vi "LCD Init by string.vi"(8 "error in":errorcluster, 11 "FPGA VI Reference In":T1) -> (0 "error out":errorcluster, 3 "FPGA VI Reference Out":T1)   [LabVIEW 2019]
uses:
  TypeDefs/FPGA Reference.ctl
  <vilib>/Utility/error.llb/Error Cluster From Error Code.vi
  <vilib>/rvi/errors/niLvFpgaAdjustHostInterfaceError.vi
  <vilib>/rvi/interface/nirviReadWriteControl/nirviReadWriteControl.xnode
  NiFpgaLv.dll
  <vilib>/rvi/interface/Simulation/niFpgaSimulationCallBeginRW.vi
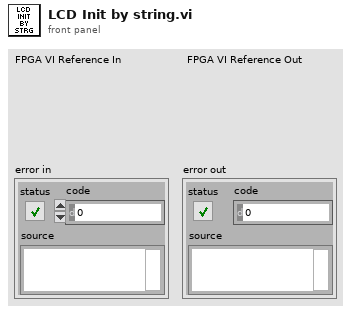
[diagram p1: front panel]
types:
  T1 = typedef "FPGA Reference.ctl" = refnum<k20>
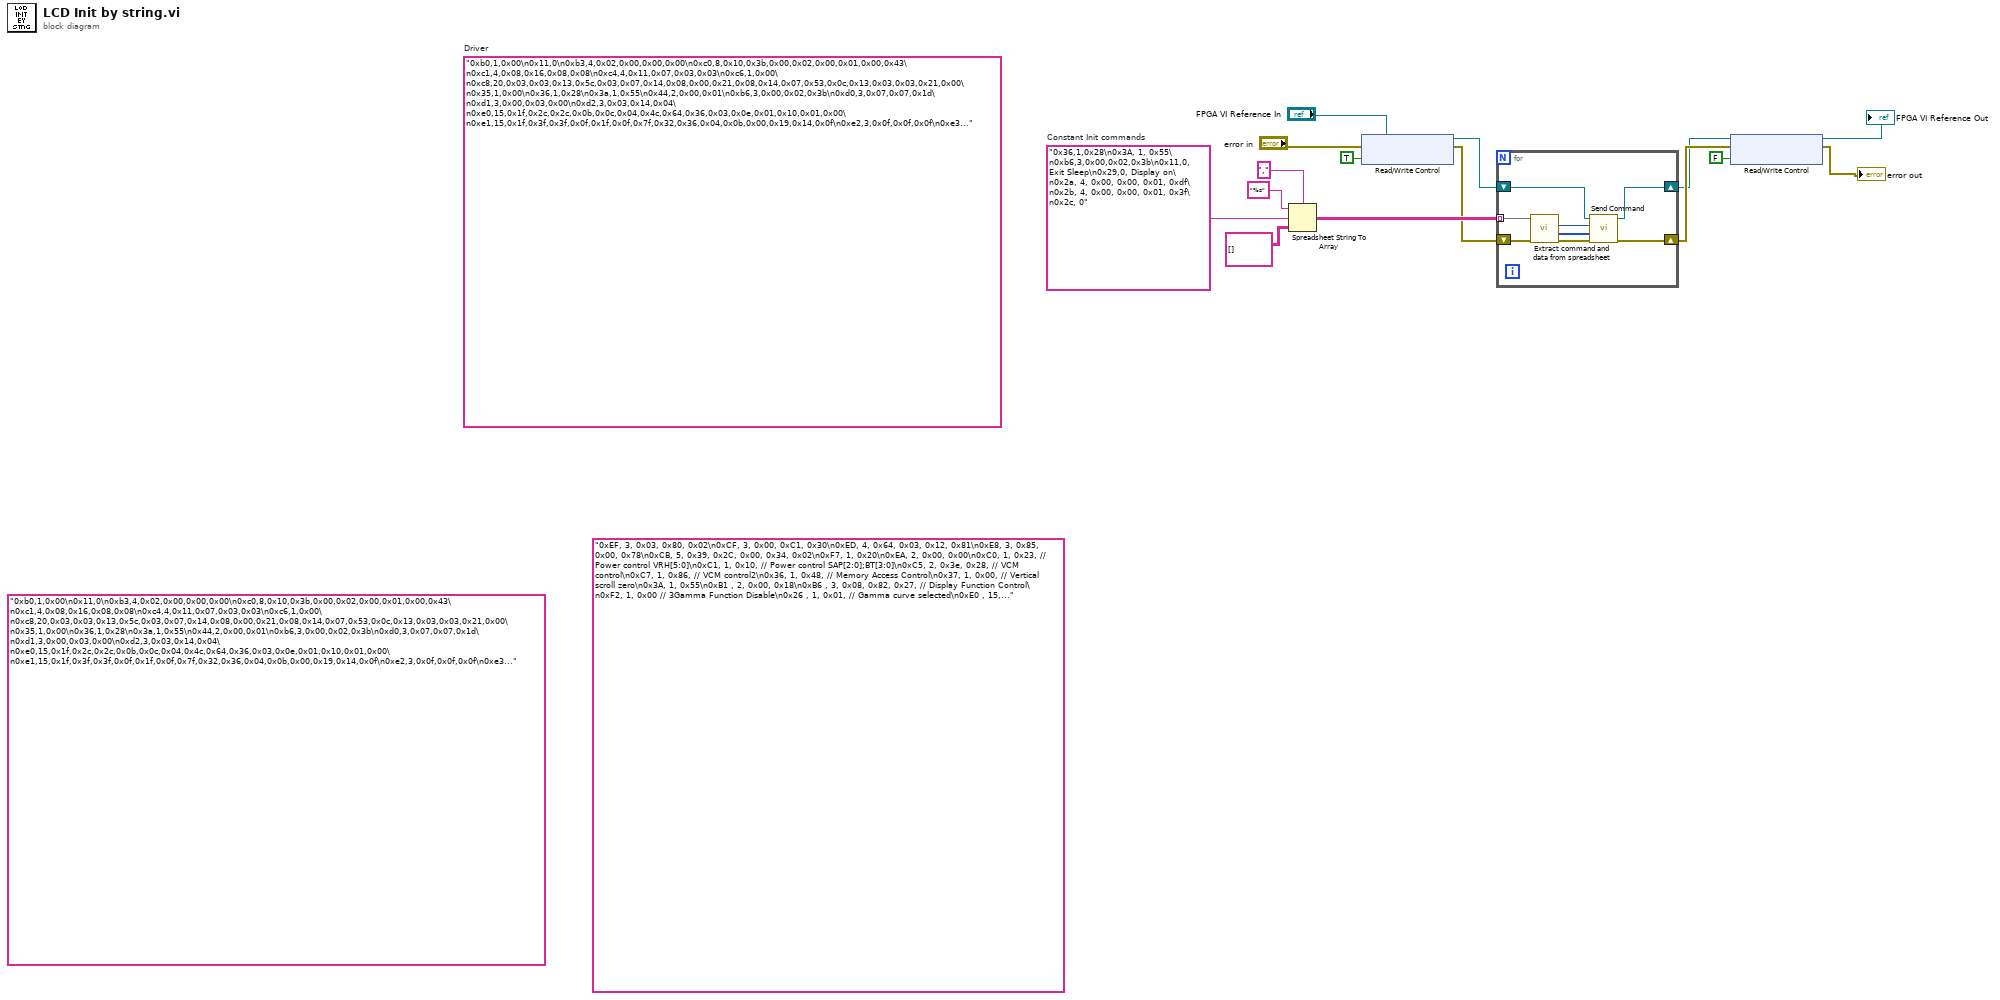
[diagram p0: block diagram]
diagram:
  w11 = "0x36,1,0x28\n0x3A, 1, 0x55\n0xb6,3,0x00,0x02,0x3b\n0x11,0, Exit Sleep\n0x29,0, Display on\n0x2a, 4, 0x00, 0x00, 0x01, 0xdf\n0x2b, 4, 0x00, 0x00, 0x01, 0x3f\n0x2c, 0"  # Constant Init commands
  (unwired) "0xEF, 3, 0x03, 0x80, 0x02\n0xCF, 3, 0x00, 0xC1, 0x30\n0xED, 4, 0x64, 0x03, 0x12, 0x81\n0xE8, 3, 0x85, 0x00, 0x78\n0xCB, 5, 0x39, 0x2C, 0x00, 0x34, 0x02\n0xF7, 1, 0x20\n0xEA, 2, 0x00, 0x00\n0xC0, 1, 0x23, // Power control VRH[5:0]\n0xC1, 1, 0x10, // Power control SAP[2:0];BT[3:0]\n0xC5, 2, 0x3e, 0x28, // VCM control\n0xC7, 1, 0x86, // VCM control2\n0x36, 1, 0x48, // Memory Access Control\n0x37, 1, 0x00, // Vertical scroll zero\n0x3A, 1, 0x55\n0xB1 , 2, 0x00, 0x18\n0xB6 , 3, 0x08, 0x82, 0x27, // Display Function Control\n0xF2, 1, 0x00 // 3Gamma Function Disable\n0x26 , 1, 0x01, // Gamma curve selected\n0xE0 , 15, 0x0F, 0x31, 0x2B, 0x0C, 0x0E, 0x08, 0x4E, 0xF1, 0x37, 0x07, 0x10, 0x03, 0x0E, 0x09, 0x00,\n0xE1 , 15, 0x00, 0x0E, 0x14, 0x03, 0x11, 0x07, 0x31, 0xC1, 0x48, 0x08, 0x0F, 0x0C, 0x31, 0x36, 0x0F\n0x11, 0x80,// Exit Sleep\n0x29, 0x80,// Display on\n0x2a, 4, 0x00, 0x00, 0x01, 0xdf\n0x2b, 4, 0x00, 0x00, 0x01, 0x3f\n0x2c, 0"
  (unwired) "0xb0,1,0x00\n0x11,0\n0xb3,4,0x02,0x00,0x00,0x00\n0xc0,8,0x10,0x3b,0x00,0x02,0x00,0x01,0x00,0x43\n0xc1,4,0x08,0x16,0x08,0x08\n0xc4,4,0x11,0x07,0x03,0x03\n0xc6,1,0x00\n0xc8,20,0x03,0x03,0x13,0x5c,0x03,0x07,0x14,0x08,0x00,0x21,0x08,0x14,0x07,0x53,0x0c,0x13,0x03,0x03,0x21,0x00\n0x35,1,0x00\n0x36,1,0x28\n0x3a,1,0x55\n0x44,2,0x00,0x01\n0xb6,3,0x00,0x02,0x3b\n0xd0,3,0x07,0x07,0x1d\n0xd1,3,0x00,0x03,0x00\n0xd2,3,0x03,0x14,0x04\n0xe0,15,0x1f,0x2c,0x2c,0x0b,0x0c,0x04,0x4c,0x64,0x36,0x03,0x0e,0x01,0x10,0x01,0x00\n0xe1,15,0x1f,0x3f,0x3f,0x0f,0x1f,0x0f,0x7f,0x32,0x36,0x04,0x0b,0x00,0x19,0x14,0x0f\n0xe2,3,0x0f,0x0f,0x0f\n0xe3,3,0x0f,0x0f,0x0f\n0x13,0\n0x29,0\n0xb4,1,0x00\n0x2xc,0\n0x2a,4,0x00,0x00,0x01,0xdf\n0x2b,4,0x00,0x00,0x01,0x3f\n0x2c,0"
  (unwired) "0xb0,1,0x00\n0x11,0\n0xb3,4,0x02,0x00,0x00,0x00\n0xc0,8,0x10,0x3b,0x00,0x02,0x00,0x01,0x00,0x43\n0xc1,4,0x08,0x16,0x08,0x08\n0xc4,4,0x11,0x07,0x03,0x03\n0xc6,1,0x00\n0xc8,20,0x03,0x03,0x13,0x5c,0x03,0x07,0x14,0x08,0x00,0x21,0x08,0x14,0x07,0x53,0x0c,0x13,0x03,0x03,0x21,0x00\n0x35,1,0x00\n0x36,1,0x28\n0x3a,1,0x55\n0x44,2,0x00,0x01\n0xb6,3,0x00,0x02,0x3b\n0xd0,3,0x07,0x07,0x1d\n0xd1,3,0x00,0x03,0x00\n0xd2,3,0x03,0x14,0x04\n0xe0,15,0x1f,0x2c,0x2c,0x0b,0x0c,0x04,0x4c,0x64,0x36,0x03,0x0e,0x01,0x10,0x01,0x00\n0xe1,15,0x1f,0x3f,0x3f,0x0f,0x1f,0x0f,0x7f,0x32,0x36,0x04,0x0b,0x00,0x19,0x14,0x0f\n0xe2,3,0x0f,0x0f,0x0f\n0xe3,3,0x0f,0x0f,0x0f\n0x13,0\n0x29,0\n0xb4,1,0x00\n0x2xc,0\n0x2a,4,0x00,0x00,0x01,0xdf\n0x2b,4,0x00,0x00,0x01,0x3f\n0x2c,0"  # Driver
  n1 = Spreadsheet String To Array(delimiter (Tab)=",", format string="%s", spreadsheet string=w11, array type (2D Dbl)=string[][] []) -> (array=w12:string[][])
  n2 = xnode "Read/Write Control"("FPGA VI Reference In"="FPGA VI Reference In", "error in"="error in", "StreamDisabled"=TRUE) -> ("FPGA VI Reference Out"=w8:T1, "error out"=w7:errorcluster)
  n3 = for {
    tunnel: w12 -> [w23] mode=indexing
    shift-right: [w21] -> w4
    shift-left: w7 -> [w19]
    shift-right: [w22] -> w3
    shift-left: w8 -> [w20]
    n4 = call "Extract command and data from spreadsheet.vi"("error in"=w19, "Data spreadsheet"=w23) -> ("error out"=w16:errorcluster, "Data"=w17:u32[], "Command"=w18:u32)  [unwired: 7 in]
    n5 = call "Send Command.vi"("error in"=w16, "Data"=w17, "Command"=w18, "FPGA VI Reference In"=w20) -> ("error out"=w21:errorcluster, "FPGA VI Reference Out"=w22:T1)  [unwired: 6 in]
  }
  n6 = xnode "Read/Write Control"("FPGA VI Reference In"=w3, "error in"=w4, "StreamDisabled"=FALSE) -> ("FPGA VI Reference Out"=→"FPGA VI Reference Out":T1, "error out"=→"error out":errorcluster)
